vi "poly_search_vis_in_memory_all.vi"(7 "app ref (open local)":refnum<vi>, 8 "error in (no error)":errorcluster) -> (0 "error out":errorcluster, 1 "vi paths":path[](array[path]), 2 "vi names":string[](array[string]), 4 "execution states":T1(array[ring]), 5 "n of vis found":i32)   [LabVIEW 2015]
doc: "Check the execution state of all VIs in the current application (or in the app reference wired <- not tested). \n\nThe target execution states are\n - \"Run Top Level\" - Runnign vi\n - \"Running\" - Running sub vi\n - \"Idle\" - Loaded in memory but not running\n - \"Bad\" - Not executable\n\nYou can use additional search items to also specity whether to search for VIs in\n - lvlibs (T)\n - llbs (T)\n - .ctl files (F)\n - reetnant instances (F)\n - this vi (F)"
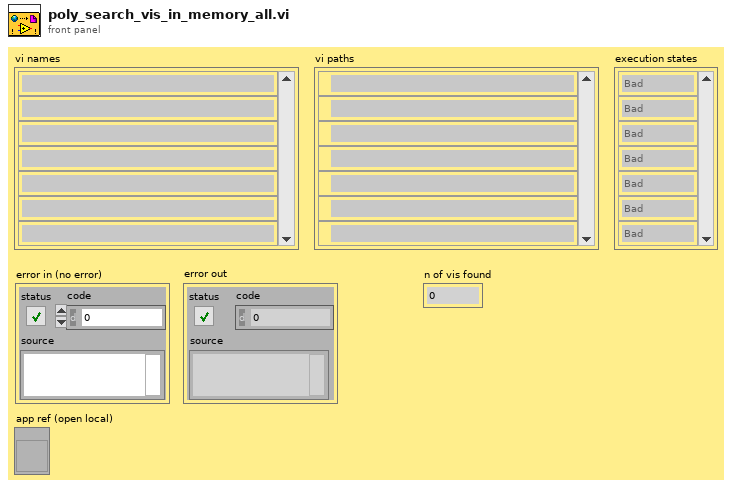
[diagram p1: front panel]
types:
  T1 = enum32{"Bad", "Idle", "Run top level", "Running"}[]
  T2 = enum32{"Bad", "Idle", "Run top level", "Running"}
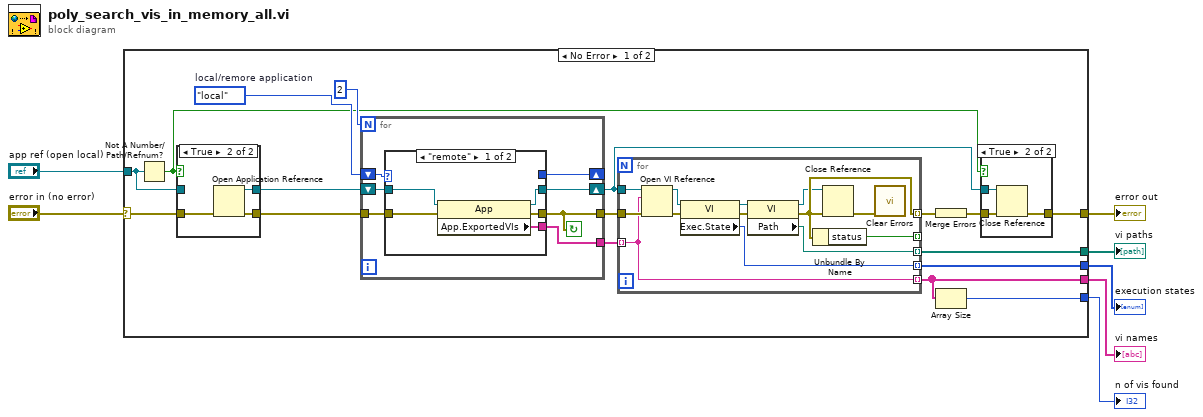
[diagram p0: block diagram]
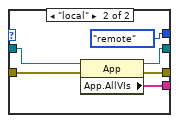
[diagram p4: hidden frame]
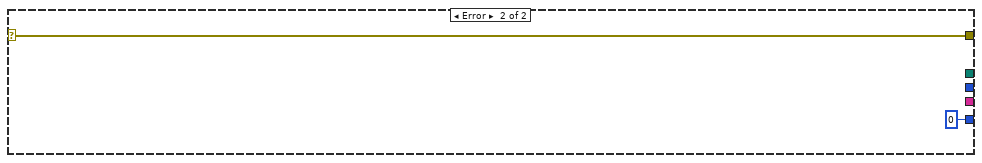
[diagram p5: hidden frame]
diagram:
  n1 = case shown="No Error" "error in (no error)" {
    selector: "error in (no error)" -> [w23 w66]
    tunnel: [w24 w66] -> w7
    tunnel: [w20 0] -> w5
    tunnel: [w22 _] -> w3
    tunnel: [w21 _] -> w4
    tunnel: "app ref (open local)" -> [w19 _]
    tunnel: [w8 _] -> w1
    frame No Error {
      w16 = enum16{"local", "remote"}."local"  # local/remore application
      n2 = Not A Number/Path/Refnum?(number/path/refnum=w19) -> (NaN/Path/Refnum?=w10:bool)
      n3 = case shown="True" w10 {
        tunnel: w23 -> [w29 w33]
        tunnel: [w30 w32] -> w15
        tunnel: [w29 w31] -> w12
        tunnel: w19 -> [w30 _]
        frame False {
        }
        frame True {
          n4 = Open Application Reference(8:w33) -> (0:w31:errorcluster, 3:w32:refnum<vi>)  [unwired: 3 in]
        }
      }
      n5 = for {
        N: 2 -> [_]
        tunnel: [w40] -> w13
        tunnel: [w39] -> w9
        shift-right: [w37] -> w14
        shift-left: w15 -> [w38]
        shift-right: [w35] -> _
        shift-left: w16 -> [w36]
        tunnel: w12 -> [w34]
        stop <- w39 continue-if-true
        n6 = case shown="\"remote\"" w36 {
          tunnel: [w44 w51] -> w40
          tunnel: [w45 w50] -> w39
          tunnel: w38 -> [w43 w47]
          tunnel: [w42 w48] -> w37
          tunnel: [_ enum16{"local", "remote"}."remote"] -> w35
          tunnel: w34 -> [w41 w46]
          frame "remote" {
            n7 = property class="App"(reference=w43, error in=w41) -> (reference out=w42:refnum<vi>, error out=w45:errorcluster, "App.ExportedVIs"=w44:string[])
          }
          frame "local" {
            n8 = property class="App"(reference=w47, error in=w46) -> (reference out=w48:refnum<vi>, error out=w50:errorcluster, "App.AllVIs"=w51:string[])
          }
        }
      }
      n9 = for {
        tunnel: w13 -> [w60] mode=indexing
        tunnel: w9 -> [w63]
        tunnel: w14 -> [w64]
        tunnel: [w53] -> w22 mode=indexing
        tunnel: [w54] -> w18 mode=indexing
        tunnel: [w61] -> _ mode=indexing
        tunnel: [w60] -> w21 mode=indexing
        tunnel: [w56] -> w8 mode=indexing
        n10 = Open VI Reference(application reference (local)=w64, vi path=w60, error in (no error)=w63) -> (vi reference=w59:refnum<vi>, error out=w57:errorcluster)  [unwired: 3 in]
        n11 = property class="VI"(reference=w59, error in=w57) -> (reference out=w58:refnum<vi>, error out=w55:errorcluster, "Exec.State"=w56:T2)
        n12 = property class="VI"(reference=w58, error in=w55) -> (reference out=w52:refnum<vi>, error out=w54:errorcluster, "Path"=w53:path)
        n13 = Unbundle By Name(w54) -> ("status"=w61:bool)
        n14 = Close Reference(reference=w52, error in (no error)=w54) -> (error out=w62:errorcluster)
        n15 = call <vilib>:"Clear Errors.vi"("error in (no error)"=w62) -> ()  [unwired: 5 in, 2 out]
      }
      n16 = Merge Errors(w18) -> (w17:errorcluster)
      n17 = Array Size(array=w21) -> (size(s)=w20:i32)
      n18 = case shown="True" w10 {
        tunnel: w17 -> [w25 w28]
        tunnel: [w25 w27] -> w24
        tunnel: w14 -> [_ w26]
        frame False {
        }
        frame True {
          n19 = Close Reference(reference=w26, error in (no error)=w28) -> (error out=w27:errorcluster)
        }
      }
    }
    frame Error {
    }
  }
  "vi names" <- w4
  "error out" <- w7
  "vi paths" <- w3
  "n of vis found" <- w5
  "execution states" <- w1
